vi "Actor Core.vi"(8 "error in":errorcluster, 11 "Filter Config Display in":refnum<class "Filter Config Display.lvclass">) -> (0 "error out":errorcluster, 3 "Actor out":refnum<class "Actor.lvclass">)   [LabVIEW 2016, in "Assert API Components.lvlib" / "Assert Display.lvlib" / "Filter Config Display.lvlib" / "Filter Config Display.lvclass"]
doc: "(<B>Filename</B>: Actor Framework.lvlib:Actor.lvclass:Actor Core.vi)\n\nReceives messages to the actor, reacts to them, and initiates any error handling that may shut the actor down.\n\nDescendant classes may override this VI to append parallel tasks for the actor to complete while it handles messages. Overrides use the Call Parent Method node."
uses:
  Filter Config Display.lvclass
  C:/Program Files (x86)/National Instruments/LabVIEW 2016/vi.lib/ActorFramework/Actor/Actor.lvclass
  D:/Work/Projects/Actor_Assert_API/Base UI Actor/Base UI Actor/Base UI Actor.lvclass
  D:/Work/Projects/Actor_Assert_API/Base UI Component/Base UI Component/Base UI Component.lvclass
  <vilib>/ActorFramework/Actor/Actor.lvclass
  Base UI Component/Base UI Component/Base UI Component.lvclass/Base UI Component.ctl
  Base UI Actor/Base UI Actor/Base UI Actor.lvclass/Base UI Actor.ctl
  <vilib>/ActorFramework/Actor/Actor.lvclass/Actor.ctl
  <vilib>/ActorFramework/Message Enqueuer/Message Enqueuer.lvclass/Message Enqueuer.ctl
  <vilib>/ActorFramework/Message Enqueuer/Init from Existing Queue.vi
  Base UI Component/Base UI Component/Base UI Component.lvclass
  <vilib>/ActorFramework/Message Enqueuer/Message Enqueuer.lvclass
  Base UI Actor/Base UI Actor/Base UI Actor.lvclass
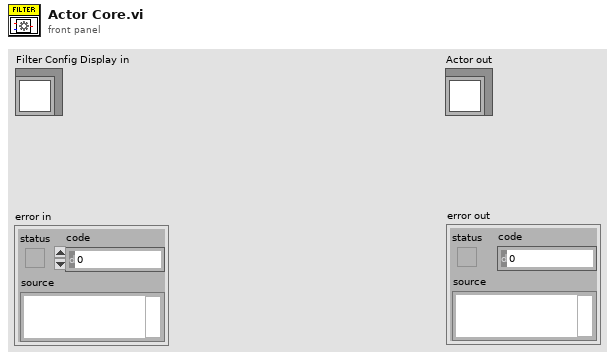
[diagram p1: front panel]
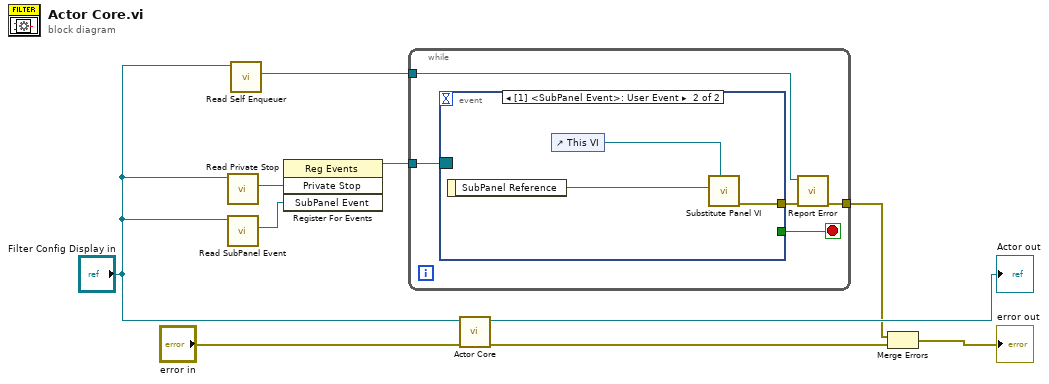
[diagram p0: block diagram]
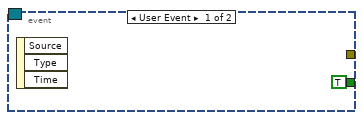
[diagram p2: hidden frame]
diagram:
  n1 = call "Read Private Stop.vi"("Base UI Actor in"="Filter Config Display in") -> ("Private Stop"=w7:refnum<user-event>)  [unwired: 10 in]
  n2 = call "Read SubPanel Event.vi"("Base UI Component in"="Filter Config Display in") -> ("SubPanel Event"=w6:refnum<user-event>)  [unwired: 10 in]
  n3 = call <vilib>:"Read Self Enqueuer.vi"("Actor"="Filter Config Display in") -> ("Self Enqueuer"=w1:refnum<class "Message Enqueuer.lvclass">)  [unwired: 10 in]
  n4 = register-events(w7, w6) -> (reference out=w5:refnum<event-registration>)  [unwired: 2 in, 1 out]
  n5 = while {
    tunnel: w5 -> [w15]
    tunnel: [w12] -> w3
    tunnel: w1 -> [w11]
    stop <- w13 stop-if-true
    n6 = event shown="[1] <SubPanel Event>: User Event" {
      selector: w15 -> [_ _]
      dyn-events: _ -> [_ _]
      timeout: _ -> [_ _]
      tunnel: [_ w19] -> w14
      tunnel: [TRUE _] -> w13
      event User Event {
        n7 = event-data() -> ()  [unwired: 1 in, 3 out]
      }
      event User Event {
        n8 = event-data() -> ("SubPanel Reference"=w18:refnum<vi>)  [unwired: 1 in]
        n9 = control-ref of="This VI"() -> (w17:refnum<vi>)
        n10 = call "Substitute Panel VI.vi"("VI Reference"=w17, "SubPanel Reference"=w18) -> ("error out"=w19:errorcluster)  [unwired: 9 in]
      }
    }
    n11 = call "Report Error.vi"("error in (no error)"=w14, "Self Enqueuer"=w11) -> ("error out"=w12:errorcluster)  [unwired: 9 in]
  }
  n12 = call-parent "Actor Core.vi"("error in"="error in", "Actor in"="Filter Config Display in") -> ("error out"=w10:errorcluster, "Actor out"=→"Actor out":refnum<class "Actor.lvclass">)  [unwired: 8 in]
  n13 = Merge Errors(w3, w10) -> (→"error out":errorcluster)
